vi "SetScanCount.vi"(8 "Error In":errorcluster, 9 "Infinite?":bool, 10 "Count (1-9999)":u32=1 min=1 max=99999 step=1, 11 "Keithley 7001 In":refnum<visa-resource-name>) -> (0 "Error Out":errorcluster, 3 "Keithley 7001 Out":refnum<visa-resource-name>)   [LabVIEW 2012, in "Keithley-7001.lvlib"]
uses:
  Keithley-7001.lvlib
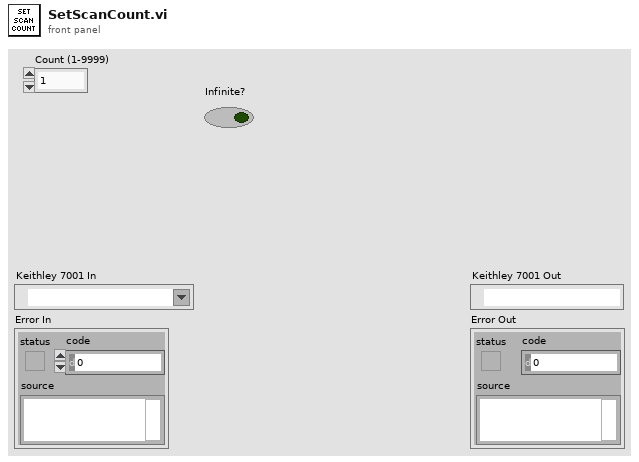
[diagram p1: front panel]
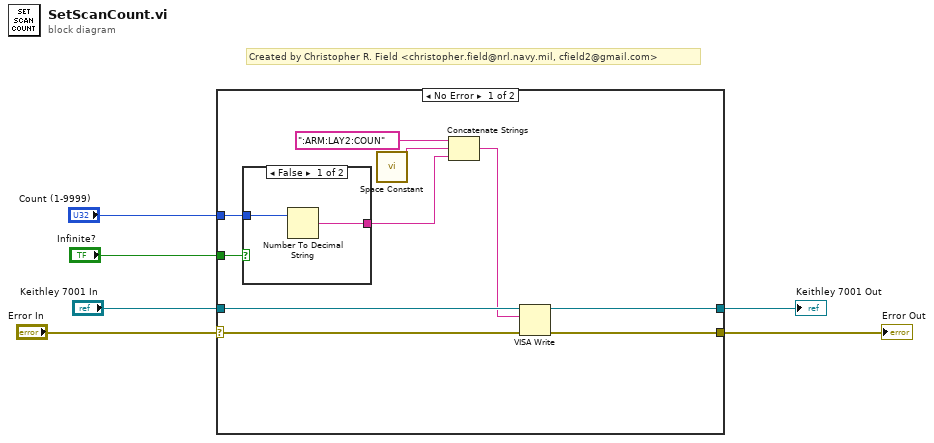
[diagram p0: block diagram]
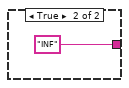
[diagram p2: hidden frame]
diagram:
  # "Created by Christopher R. Field <christopher.field@nrl.navy.mil, cfield2@gmail.com>"
  n1 = case shown="No Error" "Error In" {
    selector: "Error In" -> [w10 w20]
    tunnel: "Keithley 7001 In" -> [w16 w21]
    tunnel: [w15 w21] -> w5
    tunnel: [w14 w20] -> w4
    tunnel: "Infinite?" -> [w9 _]
    tunnel: "Count (1-9999)" -> [w7 _]
    frame No Error {
      n2 = case shown="False" w9 {
        tunnel: [w18 "INF"] -> w8
        tunnel: w7 -> [w17 _]
        frame False {
          n3 = Number To Decimal String(number=w17) -> (decimal integer string=w18:string)  [unwired: 1 in]
        }
        frame True {
        }
      }
      n4 = call <vilib>:"Space Constant.vi"() -> ("String"=w12:string)
      n5 = Concatenate Strings(":ARM:LAY2:COUN" ("write buffer"), w12, w8) -> (w11:string)
      n6 = VISA Write(VISA resource name=w16, write buffer=w11, error in (no error)=w10) -> (VISA resource name out=w15:refnum<visa-resource-name>, error out=w14:errorcluster)  [unwired: 1 out]
    }
    frame Error {
    }
  }
  "Keithley 7001 Out" <- w5
  "Error Out" <- w4
